vi "Default Instrument Setup.vi"(8 "error in (no error)":errorcluster, 10 "firmware revision":string, 11 "VISA resource name":refnum<visa-resource-name>) -> (0 "error out":errorcluster, 3 "VISA resource name out":refnum<visa-resource-name>)   [LabVIEW 2019, in "Andeen-Hagerling 2700A.lvlib"]
doc: "This Utility VI sends a default command string to the instrument whenever a new VISA session is opened, or the instrument is reset. Use this VI as a subVI for the Initialize and Reset VIs. Altering this VI could cause these two VIs to operate incorrectly."
uses:
  Andeen-Hagerling 2700A.lvlib
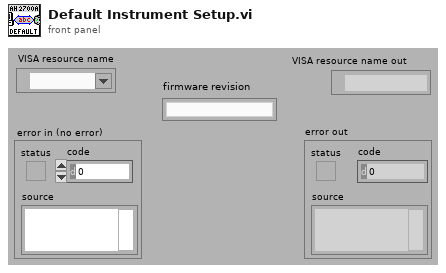
[diagram p1: front panel]
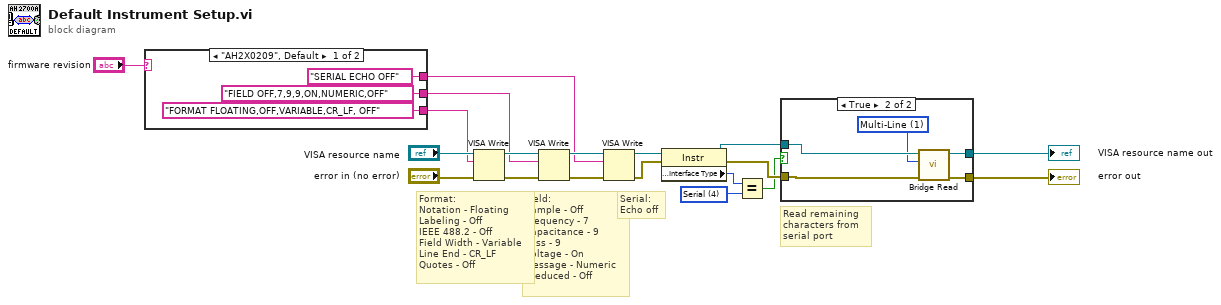
[diagram p0: block diagram]
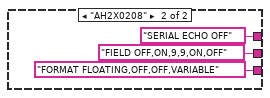
[diagram p3: hidden frame]
diagram:
  w9 = u16 4 items=["GPIB"=1, "VXI"=2, "GPIB-VXI"=3, "Serial"=4, "PXI"=5, "TCPIP"=6, "USB"=7] ("Interface Information:Interface Type")
  # "Read remaining\ncharacters from \nserial port"
  # "Serial:\nEcho off"
  # "Field:\nSample - Off\nFrequency - 7\nCapacitance - 9\nLoss - 9\nVoltage - On\nMessage - Numeric\nVreduced - Off"
  # "Format:\nNotation - Floating\nLabeling - Off\nIEEE 488.2 - Off\nField Width - Variable\nLine End - CR_LF\nQuotes - Off"
  n1 = case shown="\"AH2X0209\", Default" "firmware revision" {
    tunnel: ["FORMAT FLOATING,OFF,VARIABLE,CR_LF, OFF" "FORMAT FLOATING,OFF,OFF,VARIABLE"] -> w12
    tunnel: ["FIELD OFF,7,9,9,ON,NUMERIC,OFF" "FIELD OFF,ON,9,9,ON,OFF"] -> w11
    tunnel: ["SERIAL ECHO OFF" "SERIAL ECHO OFF"] -> w10
    frame "AH2X0209", Default {
    }
    frame "AH2X0208" {
    }
  }
  n2 = VISA Write(VISA resource name="VISA resource name", write buffer=w12, error in (no error)="error in (no error)") -> (VISA resource name out=w17:refnum<visa-resource-name>, error out=w16:errorcluster)  [unwired: 1 out]
  n3 = VISA Write(VISA resource name=w17, write buffer=w11, error in (no error)=w16) -> (VISA resource name out=w15:refnum<visa-resource-name>, error out=w14:errorcluster)  [unwired: 1 out]
  n4 = VISA Write(VISA resource name=w15, write buffer=w10, error in (no error)=w14) -> (VISA resource name out=w7:refnum<visa-resource-name>, error out=w6:errorcluster)  [unwired: 1 out]
  n5 = property class="Instr"(reference=w7, error in=w6) -> (reference out=w5:refnum<visa-resource-name>, error out=w4:errorcluster, "Interface Information:Interface Type"=w8:u16)
  n6 = Equal?(x=w8, y=w9) -> (x = y?=w3:bool)
  n7 = case shown="True" w3 {
    tunnel: w5 -> [w27 w30]
    tunnel: w4 -> [w26 w29]
    tunnel: [w27 w32] -> w2
    tunnel: [w26 w31] -> w1
    frame False {
    }
    frame True {
      w28 = u16 1 items=["Single Line", "Multi-Line"] ("Multiline")
      n8 = call "Bridge Read.vi"("error in (no error)"=w29, "multiline"=w28, "VISA resource name"=w30) -> ("error out"=w31:errorcluster, "VISA resource name out"=w32:refnum<visa-resource-name>)  [unwired: 6 in, 1 out]
    }
  }
  "error out" <- w1
  "VISA resource name out" <- w2
